vi "Parse GLL Sentence.vi"(7 "date override":timestamp format="%<%x>T", 8 "error in (no error)":errorcluster, 11 "GLL sentence":string) -> (0 "error out":errorcluster, 3 "GLL data":T1 {"type of fix"."mode" items=["Simulator", "Not Valid", "Estimated", "Differential", "Autonomous"]; "status"."value" items=["Void", "Active"]; "time of fix"."time (UTC)" format="%^<%.3X\n%x>T"})   [LabVIEW 2017, in "NMEA API.lvlib"]
doc: "Returns data contained in a particular type of NMEA sentence. The input sentence you specify must include valid NMEA formatting and end with a carriage return and line feed, or \\r\\n. You must manually select the polymorphic instance to use."
uses:
  <vilib>/robotics/Protocols/NMEA/NMEA API.lvlib
  <vilib>/robotics/Protocols/NMEA/typedefs/GLL Data.ctl
  <vilib>/robotics/Utilities/NI_Robotics Utilities.lvlib
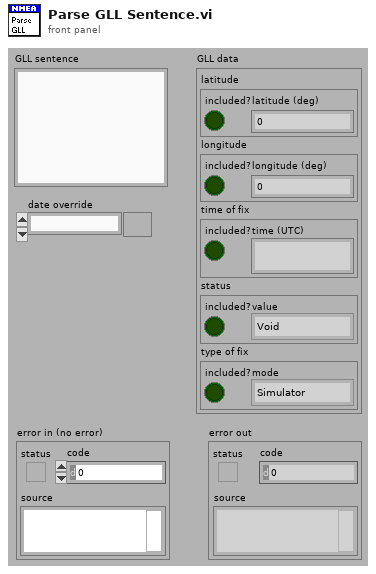
[diagram p1: front panel]
types:
  T1 = typedef "NMEA API.lvlib/GLL Data.ctl" = cluster{"latitude":cluster{"included?":bool, "latitude (deg)":dbl}, "longitude":cluster{"included?":bool, "longitude (deg)":dbl}, "time of fix":cluster{"included?":bool, "time (UTC)":timestamp}, "status":cluster{"included?":bool, "value":u16}, "type of fix":cluster{"included?":bool, "mode":u16}}
  T2 = typedef "LVDateTimeRec.ctl" = cluster{"fractional second":dbl, "second":i32, "minute":i32, "hour":i32, "day of month":i32, "month":i32, "year":i32, "day of week":i32, "day of year":i32, "DST":i32}
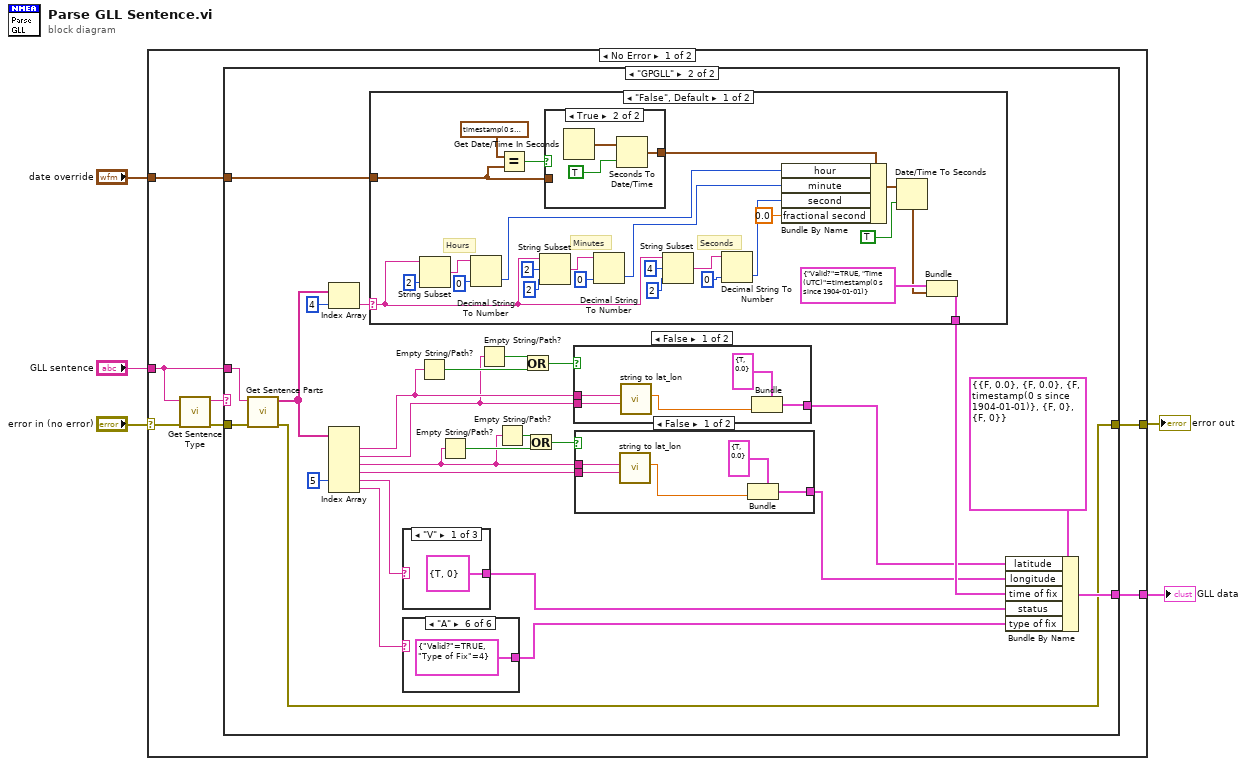
[diagram p0: block diagram]
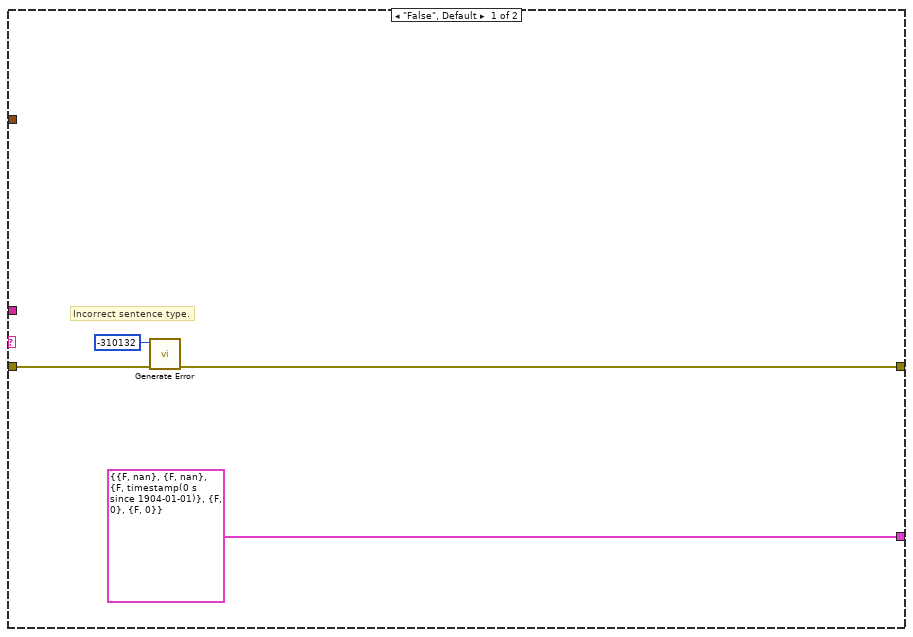
[diagram p2: hidden frame]
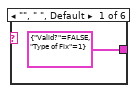
[diagram p3: hidden frame]
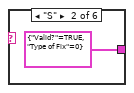
[diagram p4: hidden frame]
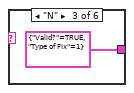
[diagram p5: hidden frame]
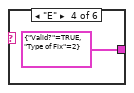
[diagram p6: hidden frame]
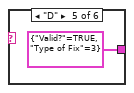
[diagram p7: hidden frame]
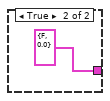
[diagram p8: hidden frame]
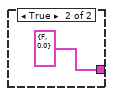
[diagram p9: hidden frame]
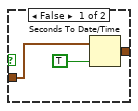
[diagram p10: hidden frame]
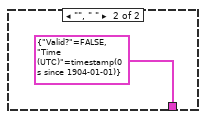
[diagram p11: hidden frame]
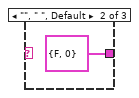
[diagram p12: hidden frame]
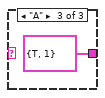
[diagram p13: hidden frame]
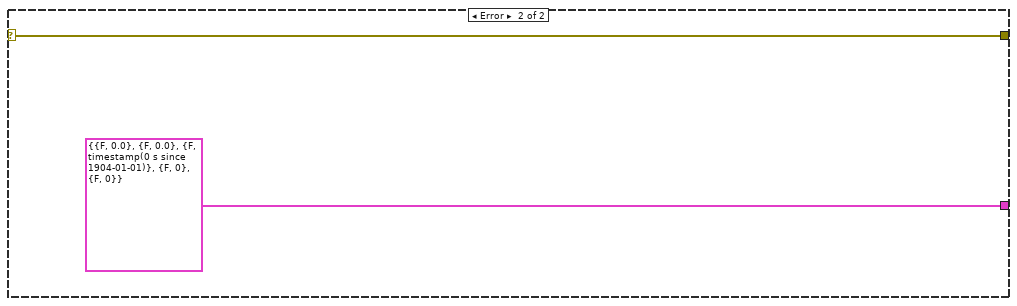
[diagram p14: hidden frame]
diagram:
  n1 = case shown="No Error" "error in (no error)" {
    selector: "error in (no error)" -> [w9 w98]
    tunnel: [w10 w98] -> w4
    tunnel: [w12 T1 {"latitude"={"included?"=FALSE, "latitude (deg)"=0.0}, "longitude"={"included?"=FALSE, "longitude (deg)"=0.0}, "time of fix"={"included?"=FALSE, "time (UTC)"=timestamp(0 s since 1904-01-01)}, "status"={"included?"=FALSE, "value"=0}, "type of fix"={"included?"=FALSE, "mode"=0}} ("GLL Data")] -> w3
    tunnel: "GLL sentence" -> [w7 _]
    tunnel: "date override" -> [w11 _]
    frame No Error {
      n2 = call <vilib>:"Get Sentence Type.vi"("error in (no error)"=w9, "sentence"=w7) -> ("error out"=w8:errorcluster, "sentence type"=w6:string)  [unwired: 1 in, 7 out]
      n3 = case shown="\"GPGLL\"" w6 {
        tunnel: w7 -> [_ w19]
        tunnel: [T1 {"latitude"={"included?"=FALSE, "latitude (deg)"=nan}, "longitude"={"included?"=FALSE, "longitude (deg)"=nan}, "time of fix"={"included?"=FALSE, "time (UTC)"=timestamp(0 s since 1904-01-01)}, "status"={"included?"=FALSE, "value"=0}, "type of fix"={"included?"=FALSE, "mode"=0}} ("GLL Data") w42] -> w12
        tunnel: w8 -> [w14 w40]
        tunnel: w11 -> [_ w30]
        tunnel: [w13 w17] -> w10
        frame "False", Default {
          # "Incorrect sentence type."
          n4 = call <vilib>:"Generate Error.vi"("error in (no error)"=w14, "code"=-310132) -> ("error out"=w13:errorcluster)  [unwired: 9 in]
        }
        frame "GPGLL" {
          n5 = call <vilib>:"Get Sentence Parts.vi"("error in (no error)"=w40, "sentence"=w19) -> ("error out"=w17:errorcluster, "sentence data"=w18:string[])  [unwired: 1 in, 7 out]
          n6 = Index Array(array=w18, index=4) -> (element=w31:string)
          n7 = Index Array(array=w18, index #5=5 ("index")) -> (element #1=w27:string, element #2=w26:string, element #3=w29:string, element #4=w28:string, element #5=w38:string, element #6=w21:string)  [unwired: 5 in]
          n8 = case shown="\"False\", Default" w31 {
            selector: w31 -> [w66 _]
            tunnel: w30 -> [w84 _]
            tunnel: [w69 cluster{"Valid?":bool, "Time (UTC)":timestamp} {"Valid?"=FALSE, "Time (UTC)"=timestamp(0 s since 1904-01-01)} ("Time of Fix")] -> w25
            frame "False", Default {
              # "Seconds"
              # "Minutes"
              # "Hours"
              n9 = String Subset(string=w66, length (rest)=2 ("length (rest)")) -> (substring=w76:string)  [unwired: 1 out]
              n10 = Decimal String To Number(string=w76, default (0L)=0 ("default (0 DBL)")) -> (number=w70:i32)  [unwired: 2 out]
              n11 = Equal?(x=timestamp(0 s since 1904-01-01), y=w84) -> (x = y?=w86:bool)
              n12 = String Subset(string=w66, offset (0)=2, length (rest)=2 ("length (rest)")) -> (substring=w77:string)
              n13 = case shown="True" w86 {
                tunnel: w84 -> [w89 _]
                tunnel: [w88 w91] -> w74
                frame False {
                  n14 = Seconds To Date/Time(time stamp (now)=w89, to UTC (F)=TRUE) -> (date time rec=w88:T2)
                }
                frame True {
                  n15 = Get Date/Time In Seconds() -> (seconds since 1Jan1904=w92:timestamp)
                  n16 = Seconds To Date/Time(time stamp (now)=w92, to UTC (F)=TRUE) -> (date time rec=w91:T2)
                }
              }
              n17 = Decimal String To Number(string=w77, default (0L)=0 ("default (0 DBL)")) -> (number=w71:i32)  [unwired: 2 out]
              n18 = String Subset(string=w66, offset (0)=4, length (rest)=2 ("length (rest)")) -> (substring=w80:string)
              n19 = Decimal String To Number(string=w80, default (0L)=0 ("default (0 DBL)")) -> (number=w72:i32)  [unwired: 2 out]
              n20 = Bundle By Name(cluster=w74, "hour"=w70, "minute"=w71, "second"=w72, "fractional second"=0.0) -> (w73:T2)
              n21 = Date/Time To Seconds(1:TRUE, 2:w73) -> (0:w67:timestamp)
              n22 = Bundle(cluster=cluster{"Valid?":bool, "Time (UTC)":timestamp} {"Valid?"=TRUE, "Time (UTC)"=timestamp(0 s since 1904-01-01)} ("Time of Fix"), "Time (UTC)"=w67) -> (w69:cluster{"Valid?":bool, "Time (UTC)":timestamp})  [unwired: 1 out]
            }
            frame "", " " {
            }
          }
          n23 = case shown="\"V\"" w38 {
            tunnel: [cluster{"Valid?":bool, "Status":u16} {"Valid?"=TRUE, "Status"=0} ("Status") cluster{"Valid?":bool, "Status":u16} {"Valid?"=FALSE, "Status"=0} ("Status") cluster{"Valid?":bool, "Status":u16} {"Valid?"=TRUE, "Status"=1} ("Status")] -> w22
            frame "V" {
            }
            frame "", " ", Default {
            }
            frame "A" {
            }
          }
          n24 = case shown="\"A\"" w21 {
            tunnel: [cluster{"Valid?":bool, "Type of Fix":u16} {"Valid?"=FALSE, "Type of Fix"=1} ("Type of Fix") cluster{"Valid?":bool, "Type of Fix":u16} {"Valid?"=TRUE, "Type of Fix"=0} ("Type of Fix") cluster{"Valid?":bool, "Type of Fix":u16} {"Valid?"=TRUE, "Type of Fix"=1} ("Type of Fix") cluster{"Valid?":bool, "Type of Fix":u16} {"Valid?"=TRUE, "Type of Fix"=2} ("Type of Fix") cluster{"Valid?":bool, "Type of Fix":u16} {"Valid?"=TRUE, "Type of Fix"=3} ("Type of Fix") cluster{"Valid?":bool, "Type of Fix":u16} {"Valid?"=TRUE, "Type of Fix"=4} ("Type of Fix")] -> w20
            frame "", " ", Default {
            }
            frame "S" {
            }
            frame "N" {
            }
            frame "E" {
            }
            frame "D" {
            }
            frame "A" {
            }
          }
          n25 = Empty String/Path?(string/path=w27) -> (empty?=w35:bool)
          n26 = Empty String/Path?(string/path=w29) -> (empty?=w34:bool)
          n27 = Empty String/Path?(string/path=w26) -> (empty?=w36:bool)
          n28 = Empty String/Path?(string/path=w29) -> (empty?=w33:bool)
          n29 = Or(x=w36, y=w35) -> (x .or. y?=w37:bool)
          n30 = Or(x=w33, y=w34) -> (x .or. y?=w32:bool)
          n31 = case shown="False" w37 {
            tunnel: [w58 cluster{"Valid?":bool, "Latitude (Deg)":dbl} {"Valid?"=FALSE, "Latitude (Deg)"=0.0} ("Latitude")] -> w24
            tunnel: w27 -> [w60 _]
            tunnel: w26 -> [w59 _]
            frame False {
              n32 = call <vilib>:"string to lat_lon.vi"("direction string"=w59, "numeric string for lat/lon"=w60) -> ("composite value"=w56:dbl)  [unwired: 1 in, 8 out]
              n33 = Bundle(cluster=cluster{"Valid?":bool, "Latitude (Deg)":dbl} {"Valid?"=TRUE, "Latitude (Deg)"=0.0} ("Latitude"), "Latitude (Deg)"=w56) -> (w58:cluster{"Valid?":bool, "Latitude (Deg)":dbl})  [unwired: 1 out]
            }
            frame True {
            }
          }
          n34 = case shown="False" w32 {
            tunnel: w28 -> [w54 _]
            tunnel: w29 -> [w53 _]
            tunnel: [w50 cluster{"Valid?":bool, "Longitude (Deg)":dbl} {"Valid?"=FALSE, "Longitude (Deg)"=0.0} ("Longitude")] -> w23
            frame False {
              n35 = call <vilib>:"string to lat_lon.vi"("direction string"=w54, "numeric string for lat/lon"=w53) -> ("composite value"=w52:dbl)  [unwired: 1 in, 8 out]
              n36 = Bundle(cluster=cluster{"Valid?":bool, "Longitude (Deg)":dbl} {"Valid?"=TRUE, "Longitude (Deg)"=0.0} ("Longitude"), "Longitude (Deg)"=w52) -> (w50:cluster{"Valid?":bool, "Longitude (Deg)":dbl})  [unwired: 1 out]
            }
            frame True {
            }
          }
          n37 = Bundle By Name(cluster=T1 {"latitude"={"included?"=FALSE, "latitude (deg)"=0.0}, "longitude"={"included?"=FALSE, "longitude (deg)"=0.0}, "time of fix"={"included?"=FALSE, "time (UTC)"=timestamp(0 s since 1904-01-01)}, "status"={"included?"=FALSE, "value"=0}, "type of fix"={"included?"=FALSE, "mode"=0}} ("GLL Data"), "latitude"=w24, "longitude"=w23, "time of fix"=w25, "status"=w22, "type of fix"=w20) -> (w42:T1)
        }
      }
    }
    frame Error {
    }
  }
  "error out" <- w4
  "GLL data" <- w3
